vi "Teardown for Get File Content.vi"(8 "error in (no error)":errorcluster, 11 "read file.lvclass":refnum<class "read file.lvclass">) -> (0 "error out":errorcluster)   [LabVIEW 2017]
doc: "The reference number from Read File Refnum VI passes to this VI. Use this VI as a teardown VI for the Get File Content.lvtest test."
uses:
  read file.lvclass
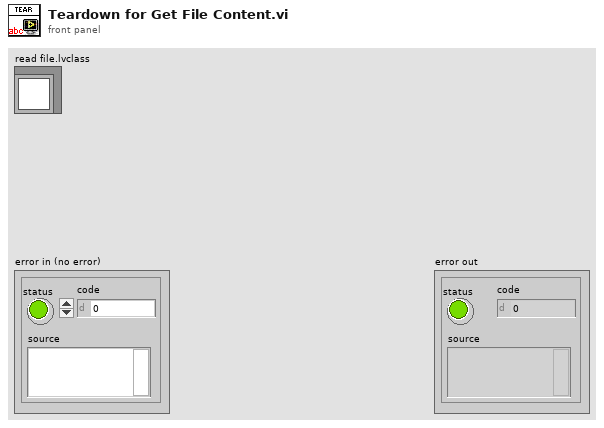
[diagram p1: front panel]
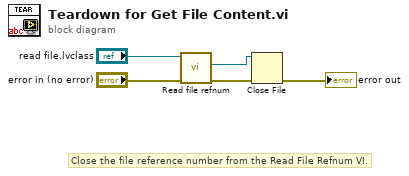
[diagram p0: block diagram]
diagram:
  # "Close the file reference number from the Read File Refnum VI."
  n1 = call "Read file refnum.vi"("error in (no error)"="error in (no error)", "read file in"="read file.lvclass") -> ("error out"=w3:errorcluster, "file refnum"=w2:refnum<file>)  [unwired: 7 in, 1 out]
  n2 = Close File(refnum=w2, error in=w3) -> (error out=→"error out":errorcluster)  [unwired: 1 out]
